vi "commit configurations and build.vi"(8 "error in (no error)":errorcluster, 10 "version":T1, 11 "NI_AB_API_PPL in":refnum<class "NI_AB_API_PPL.lvclass">) -> (0 "error out":errorcluster, 2 "Destinations":T2[](array[typedef]), 3 "GeneratedFiles":path[](array[path]))   [LabVIEW 2024]
uses:
  <vilib>/AppBuilder/AB_API/common/AB_API Destination Type.ctl
  <vilib>/AppBuilder/AB_API/common/AB_API Destination Data.ctl
  <vilib>/AppBuilder/AB_API/PPL/NI_AB_API_PPL.lvclass
  <vilib>/AppBuilder/AB_API/common/AB_API Version Number.ctl
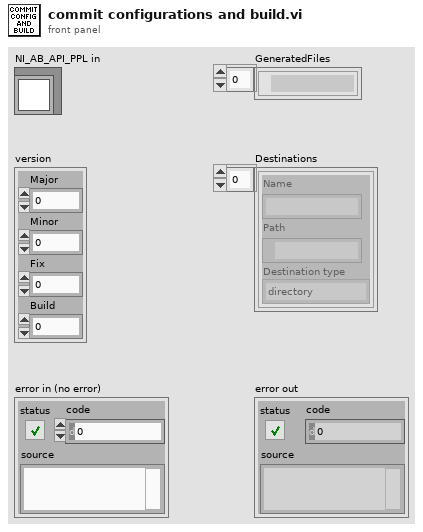
[diagram p1: front panel]
types:
  T1 = typedef "AB_API Version Number.ctl" = cluster{"Major":u16, "Minor":u16, "Fix":u16, "Build":u16}
  T2 = typedef "AB_API Destination Data.ctl" = cluster{"Name":string, "Path":path, "Destination type":T3}
  T3 = typedef "AB_API Destination Type.ctl" = enum16{"directory", "directory (preserve hierarchy)", "LLB"}
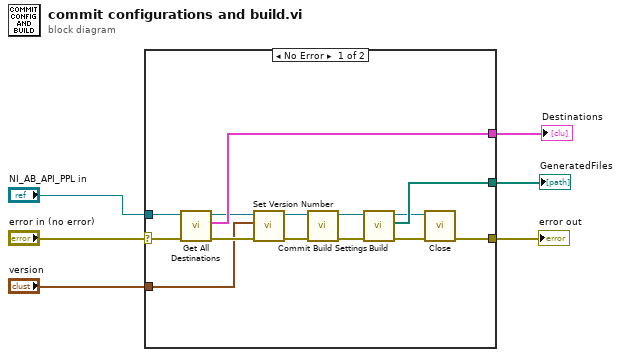
[diagram p0: block diagram]
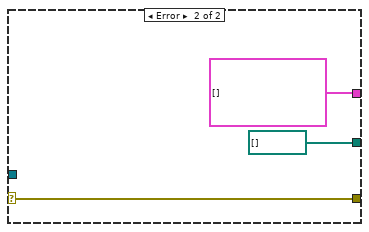
[diagram p2: hidden frame]
diagram:
  n1 = case shown="No Error" "error in (no error)" {
    selector: "error in (no error)" -> [w16 w23]
    tunnel: [w20 w23] -> w6
    tunnel: [w19 T2[] [] ("Destinations")] -> w5
    tunnel: "NI_AB_API_PPL in" -> [w15 _]
    tunnel: "version" -> [w14 _]
    tunnel: [w11 path[] [] ("GeneratedFiles")] -> w1
    frame No Error {
      n2 = call-dynamic "Get All Destinations.vi"("error in (no error)"=w16, "NI_AB_API_Build in"=w15) -> ("error out"=w17:errorcluster, "Destinations"=w19:T2[], "NI_AB_API_Build out"=w18:refnum<class "NI_AB_API_PPL.lvclass">)  [unwired: 7 in]
      n3 = call-dynamic "Set Version Number.vi"("error in (no error)"=w17, "Version number"=w14, "PPL in"=w18) -> ("error out"=w12:errorcluster, "PPL out"=w13:refnum<class "NI_AB_API_PPL.lvclass">)  [unwired: 7 in]
      n4 = call-dynamic "Commit Build Settings.vi"("error in (no error)"=w12, "PPL in"=w13) -> ("error out"=w7:errorcluster, "PPL out"=w9:refnum<class "NI_AB_API_PPL.lvclass">)  [unwired: 8 in]
      n5 = call-dynamic "Build.vi"("error in (no error)"=w7, "PPL in"=w9) -> ("error out"=w8:errorcluster, "GeneratedFiles"=w11:path[], "PPL out"=w10:refnum<class "NI_AB_API_PPL.lvclass">)  [unwired: 6 in, 1 out]
      n6 = call-dynamic "Close.vi"("error in (no error)"=w8, "DLL in"=w10) -> ("error out"=w20:errorcluster)  [unwired: 9 in]
    }
    frame Error {
    }
  }
  "error out" <- w6
  "Destinations" <- w5
  "GeneratedFiles" <- w1
